vi "basic - VL Receive.vi"() -> ()   [LabVIEW 2020]
uses:
  src/_polimorphicInstances/session/Fdx Close Session (Port).vi
  src/AIM664LV.lvlib
  <extravilib>/ChannelInstances/Tag-bool.lvlib
  src/_polimorphicInstances/session/Fdx Create Session (Rx-VL-Oriented).vi
  src/bsp/AFDX_Receive/Fdx Create Rx VL.vi
  src/_polimorphicInstances/udpPort/Fdx Create UDP Port (RX-CommPort).vi
  src/_polimorphicInstances/control/Fdx Start (Rx).vi
  src/_polimorphicInstances/control/Fdx Stop (Rx).vi
  src/_controls/comm_computedMAC-IP.ctl
  src/_controls/comm_verification_rx.ctl
  src/_controls/comm_udp_rx.ctl
panel:
  in  "DefaultPayloadMode (Full)":u32(ring) items=["FDX_PAYLOAD_FULL", "FDX_PAYLOAD_IP_EXT", "FDX_PAYLOAD_IP", "FDX_PAYLOAD_MAC"]
  in  "Board":u32
  in  "Port":u32=1
  out "CommPort Addresses":T1[](array[typedef])=[{"MACsrc"=[], "IPsrc"="10.1.33.1", "IPdest"="224.224.0.60"}, {"MACsrc"=[], "IPsrc"="10.1.33.1", "IPdest"="224.224.0.60"}] {"MACsrc" format="%.0x"}
  in  "VL Config":T2={"VlId"=60, "VLRange"=2, "VerificationMode"=0, "Bag"=0, "Jitter"=0, "MaxFrameLength"=0, "MaxSkew"=0, "VLBufSize"=32768, "FilterMode"=0, "FilterPosition"=0, "Padding"=0, "FilterMask"=0, "FilterData"=0, "MinFrameLength"=0} {"FilterMode" items=["FDX_RX_VL_FLT_DIS", "FDX_RX_VL_FLT_ENA ", "FDX_RX_VL_FLT_ENA_INV"]; "MaxFrameLength" format="%.0x"; "VerificationMode" items=["FDX_RX_VL_CHECK_ENA_DEFAULT"=65535, "FDX_RX_VL_CHECK_REDMAM"=16, "DX_RX_VL_CHECK_TRAFIC"=8, "FDX_RX_VL_CHECK_FRAMESIZE"=4, "FDX_RX_VL_CHECK_SNINTEG"=2, "FDX_RX_VL_CHECK_INVPAC"=1, "FDX_RX_VL_CHECK_DISA"=0]}
  in  "CommPort Config":T3[](array[typedef])=[{"PortType"=enum."FDX_UDP_SAMPLING", "SubVIId"=1, "domainID"=1, "sideID"=1, "locationID"=1, "partitionID"=1, "UdpSrcPort"=1, "UdpDstPort"=1, "UdpNumBufMessages"=1, "UdpMaxMessageSize"=1000, "UdpSamplingRate"=0}, {"PortType"=enum."FDX_UDP_SAMPLING", "SubVIId"=2, "domainID"=1, "sideID"=1, "locationID"=1, "partitionID"=1, "UdpSrcPort"=2, "UdpDstPort"=2, "UdpNumBufMessages"=1, "UdpMaxMessageSize"=1000, "UdpSamplingRate"=0}] {"partitionID" format="%.0b"}
  out "read time uS":u32(graph)=3177
  in  "poll rate mS 1":u32=10
  out "data":cluster{"Data":u8[]}[](array[cluster])
  out "BytesRead":u32[](array[numeric])
  out "current time":timestamp=timestamp(3686488955.9671674 s since 1904-01-01)
  out "current irig time":T4={"SignOut"=-1509901600, "DayOut"=16, "HourOut"=8, "MinOut"=7, "SecondOut"=53, "MilliSecOut"=368, "MicroSecOut"=508, "NanoSecOut"=600, "InfoOut"=0, "Mode"=3}
  in  "stop":bool
  out "PortInitOut":T5={"PortConfig"=0, "PortUsed"=1, "GlobalMemFree"=0, "SharedMemFree"=0} {"PortConfig" items=["FDX_SINGLE", "FDX_REDUNDANT"]}
  out "error out":errorcluster
  # "ARINC 664 - Receiving through VL (Virtual Link)"
  # "Overview: Setup the board to transmit package as raw frames.\nRequirement: One AIM ARINC-664 board with installed AIM ARINC 664 BSP.\nRestrictions: None.\nInstruction:\n1. Select the Board ID (0 if you have only one board in your system) and the port number. If you want to validate between two ports in one device, you can use tx board and Rx Board\n2. Run the VI.\n3. See the result in Current IRIG Time"
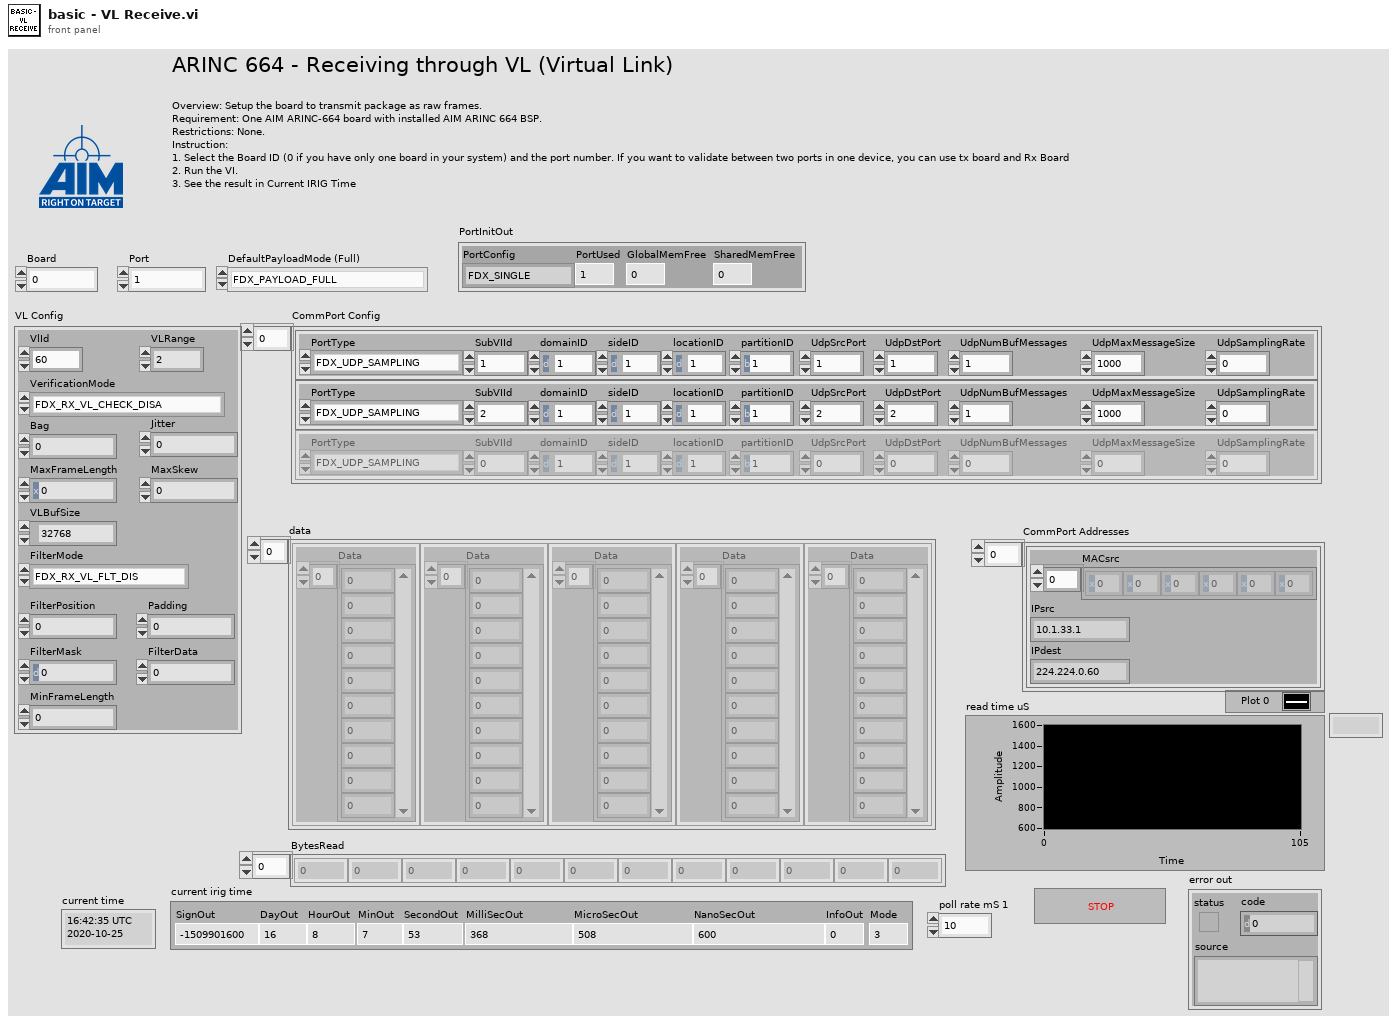
[diagram p1: front panel]
types:
  T1 = typedef "AIM664LV.lvlib/comm_computedMAC-IP.ctl" = cluster{"MACsrc":u8[], "IPsrc":string, "IPdest":string}
  T2 = typedef "AIM664LV.lvlib/comm_verification_rx.ctl" = cluster{"VlId":u16, "VLRange":u32, "VerificationMode":u32, "Bag":u32, "Jitter":u32, "MaxFrameLength":u32, "MaxSkew":u32, "VLBufSize":u32, "FilterMode":u32, "FilterPosition":u32, "Padding":u32, "FilterMask":u32, "FilterData":u32, "MinFrameLength":u32}
  T3 = typedef "AIM664LV.lvlib/comm_udp_rx.ctl" = cluster{"PortType":enum16{"FDX_UDP_SAMPLING", "FDX_UDP_QUEUING"}, "SubVIId":u32, "domainID":u8, "sideID":u8, "locationID":u8, "partitionID":u8, "UdpSrcPort":u16, "UdpDstPort":u16, "UdpNumBufMessages":u32, "UdpMaxMessageSize":u32, "UdpSamplingRate":u32}
  T4 = cluster{"SignOut":i32, "DayOut":u32, "HourOut":u32, "MinOut":u32, "SecondOut":u32, "MilliSecOut":u32, "MicroSecOut":u32, "NanoSecOut":u32, "InfoOut":u32, "Mode":u32}
  T5 = cluster{"PortConfig":u32, "PortUsed":u32, "GlobalMemFree":u32, "SharedMemFree":u32}
  T6 = typedef "Tag-bool.lvlib/))Channel.ctl" = refnum<queue>
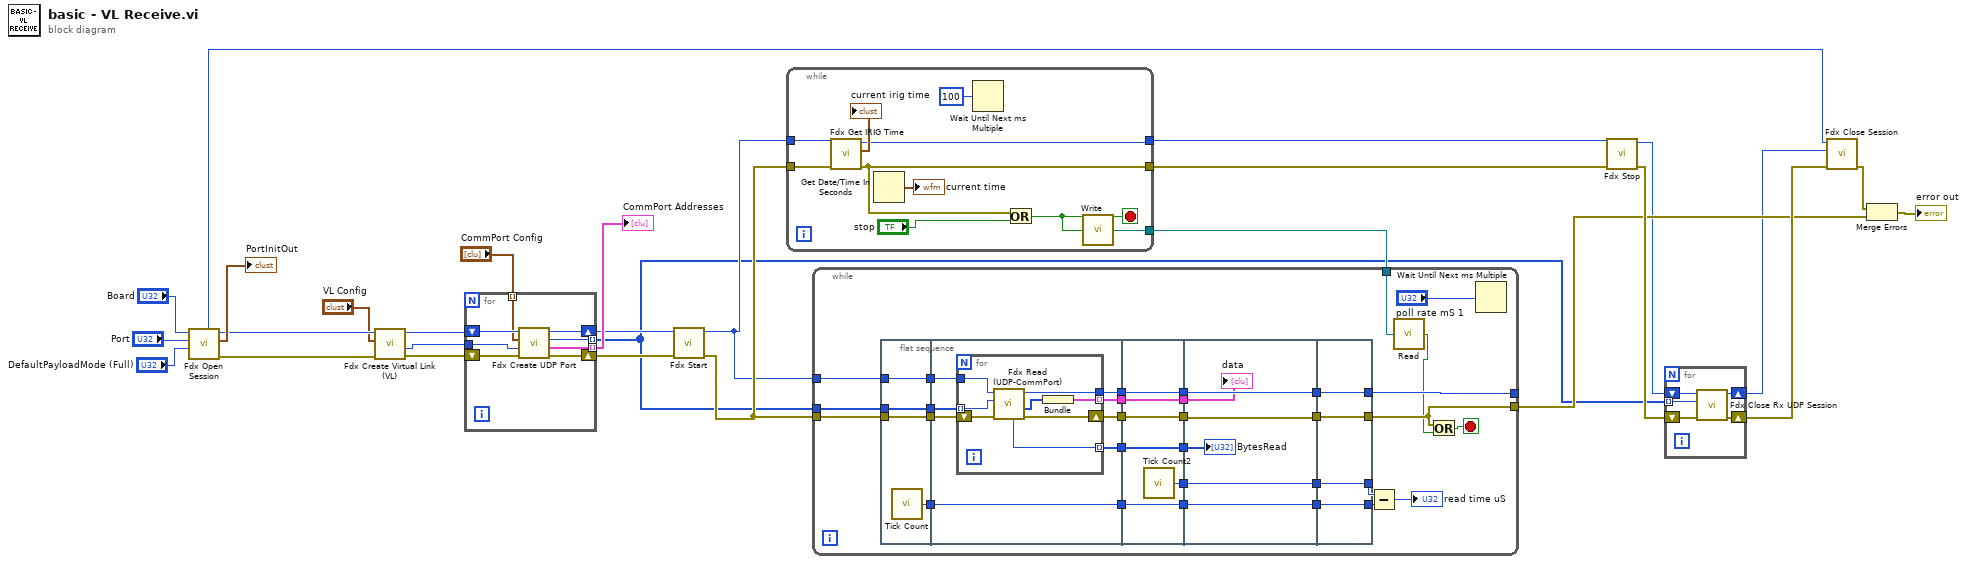
[diagram p0: block diagram]
diagram:
  n1 = call-poly "Fdx Open Session.vi"("DefaultPayloadMode (Full)"="DefaultPayloadMode (Full)", "port"="Port", "board"="Board") -> ("error out"=w12:errorcluster, "PortInitOut"=→"PortInitOut":T5, "InstrumentHandle_port out"=w13:u32, "InstrumentHandle_board out"=w1:u32)  [unwired: 3 in, 2 out]
  n2 = call-poly "Fdx Create Virtual Link (VL).vi"("error in (no error)"=w12, "VL Config"="VL Config", "InstrumentHandle_port in"=w13) -> ("error out"=w9:errorcluster, "VlId"=w8:u16, "InstrumentHandle_port out"=w10:u32)  [unwired: 6 in]
  n3 = for {
    tunnel: [w35] -> w27 mode=indexing
    tunnel: [w31] -> w2 mode=indexing
    shift-right: [w36] -> w28
    shift-left: w9 -> [w33]
    shift-right: [w34] -> w26
    shift-left: w10 -> [w32]
    tunnel: w8 -> [w30]
    tunnel: "CommPort Config" -> [w29] mode=indexing
    n4 = call-poly "Fdx Create UDP Port.vi"("error in (no error)"=w33, "VlId"=w30, "CommPort Config"=w29, "port handle in"=w32) -> ("error out"=w36:errorcluster, "computedAddresses"=w35:T1, "commPort handle out"=w31:u32, "port handle out"=w34:u32)  [unwired: 4 in]
  }
  "CommPort Addresses" <- w27
  n5 = call-poly "Fdx Start.vi"("error in (no error)"=w28, "InstrumentHandle_port in"=w26) -> ("error out"=w19:errorcluster, "InstrumentHandle_port out"=w3:u32)  [unwired: 8 in]
  n6 = while {
    tunnel: w3 -> [w45]
    tunnel: w19 -> [w44]
    tunnel: [w42] -> w22
    tunnel: [w41] -> w21
    tunnel: [w37] -> w17
    stop <- w38 stop-if-true
    n7 = call "Fdx Get IRIG Time.vi"("error in (no error)"=w44, "InstrumentHandle_board in"=w45) -> ("error out"=w41:errorcluster, "Curent Irig Time"=→"current irig time":T4, "InstrumentHandle_board out"=w42:u32)  [unwired: 7 in]
    n8 = Get Date/Time In Seconds() -> (seconds since 1Jan1904=→"current time":timestamp)
    n9 = Wait Until Next ms Multiple(millisecond multiple=u32 100) -> ()  [unwired: 1 out]
    n10 = Or(x=w41, y="stop") -> (x .or. y?=w38:bool)
    n11 = call <extravilib>:"Write.vi"("element"=w38) -> ("channel"=w37:T6)  [unwired: 1 out]
  }
  n12 = while {
    tunnel: w19 -> [w76]
    tunnel: w2 -> [w75]
    tunnel: [w63] -> _
    tunnel: [w56] -> w14
    tunnel: w17 -> [w51]
    tunnel: w3 -> [w48]
    stop <- w77 stop-if-true
    n13 = flat-sequence {
      tunnel: w76 -> [w80]
      tunnel: w75 -> [w81]
      tunnel: [w81] -> w71
      tunnel: [w80] -> w70
      tunnel: [w79] -> w69
      tunnel: w48 -> [w78]
      tunnel: [w78] -> w47
      tunnel: w71 -> [w83]
      tunnel: w70 -> [w89]
      tunnel: w69 -> [w88]
      tunnel: [w88] -> w68
      tunnel: [w87] -> w60
      tunnel: [w86] -> w57
      tunnel: [w85] -> w54
      tunnel: [w84] -> w52
      tunnel: w47 -> [w82]
      tunnel: w68 -> [w103]
      tunnel: [w103] -> w67
      tunnel: [w102] -> w64
      tunnel: [w101] -> w61
      tunnel: w60 -> [w101]
      tunnel: [w100] -> w58
      tunnel: w57 -> [w100]
      tunnel: [w99] -> w55
      tunnel: w54 -> [w99]
      tunnel: [w98] -> w53
      tunnel: w52 -> [w98]
      tunnel: w67 -> [w109]
      tunnel: [w109] -> w73
      tunnel: [w108] -> w65
      tunnel: w64 -> [w108]
      tunnel: [w107] -> w62
      tunnel: w61 -> [w107]
      tunnel: [w106] -> w59
      tunnel: w58 -> [w106]
      tunnel: w55 -> [w104]
      tunnel: w53 -> [w105]
      tunnel: [w113] -> w74
      tunnel: w73 -> [w113]
      tunnel: [w112] -> w66
      tunnel: w65 -> [w112]
      tunnel: [w111] -> w63
      tunnel: w62 -> [w111]
      tunnel: [w110] -> w56
      tunnel: w59 -> [w110]
      frame #0 {
        n14 = call "Tick Count"() -> ("Tick Count(uSec)"=w79:u32)
      }
      frame #1 {
        n15 = for {
          tunnel: [w96] -> w87
          tunnel: [w90] -> w85 mode=indexing
          tunnel: [w94] -> w84 mode=indexing
          tunnel: w83 -> [w93] mode=indexing
          tunnel: w82 -> [w92]
          shift-right: [w95] -> w86
          shift-left: w89 -> [w97]
          n16 = call "Fdx Read (UDP-CommPort).vi"("error in (no error)"=w97, "UdpHandle in"=w93, "InstrumentHandle_port in"=w92) -> ("error out"=w95:errorcluster, "Data"=w91:u8[], "InstrumentHandle_port out"=w96:u32, "MsgRead"=w94:u32)  [unwired: 4 in, 1 out]
          n17 = Bundle("Data"=w91) -> (w90:cluster{"Data":u8[]})  [unwired: 1 in]
        }
      }
      frame #2 {
        n18 = call "Tick Count2"() -> ("Tick Count(uSec)"=w102:u32)
      }
      frame #3 {
        "BytesRead" <- w105
        "data" <- w104
      }
      frame #4 {
      }
    }
    n19 = Subtract(x=w66, y=w74) -> (x-y=→"read time uS":u32)
    n20 = call <extravilib>:"Read.vi"("channel"=w51) -> ("element"=w50:bool)  [unwired: 1 in, 1 out]
    n21 = Or(x=w56, y=w50) -> (x .or. y?=w77:bool)
    n22 = Wait Until Next ms Multiple(millisecond multiple="poll rate mS 1") -> ()  [unwired: 1 out]
  }
  n23 = call-poly "Fdx Stop.vi"("error in (no error)"=w21, "InstrumentHandle_port in"=w22) -> ("error out"=w20:errorcluster, "InstrumentHandle_port out"=w5:u32)  [unwired: 8 in]
  n24 = for {
    tunnel: w2 -> [w114] mode=indexing
    shift-right: [w117] -> w18
    shift-left: w20 -> [w118]
    shift-right: [w115] -> w4
    shift-left: w5 -> [w116]
    n25 = call "Fdx Close Rx UDP Session.vi"("error in (no error)"=w118, "UdpHandle in"=w114, "InstrumentHandle_port in"=w116) -> ("error out"=w117:errorcluster, "InstrumentHandle_port out"=w115:u32)  [unwired: 7 in]
  }
  n26 = call-poly "Fdx Close Session.vi"("error in (no error)"=w18, "InstrumentHandle_port in"=w4, "InstrumentHandle_board in"=w1) -> ("error out"=w16:errorcluster)  [unwired: 8 in]
  n27 = Merge Errors(w16, w14) -> (→"error out":errorcluster)
